vi "Find Device by Listbox Value.vi"(3 "error in (no error)":errorcluster, 4 "Listbox":refnum<vi>, 5 "ACNET Devices":refnum<class "ACNET Devices.lvclass">) -> (0 "error out":errorcluster, 1 "Found?":bool, 2 "ACNET Device Cluster":T1)   [LabVIEW 2013, in "ACNET Monitor.lvlib"]
uses:
  ACNET Monitor.lvlib
  ACNET Devices.lvclass
  ACNET Device.lvclass
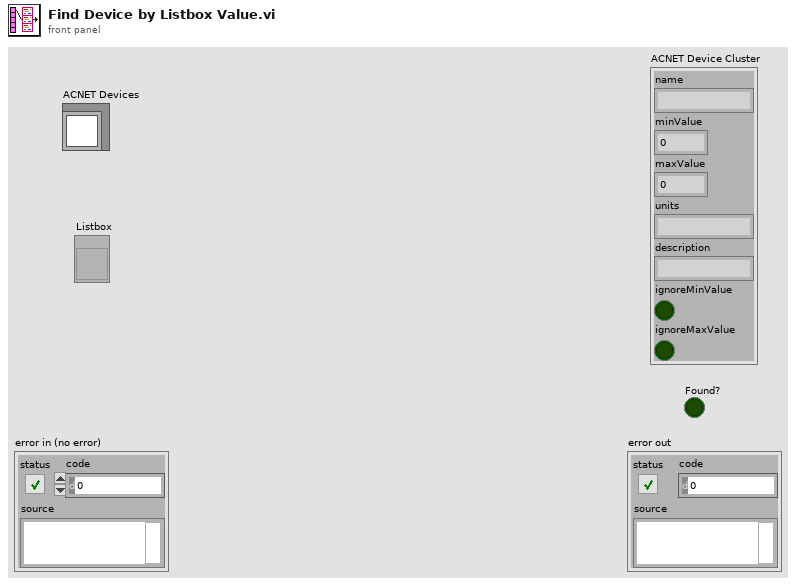
[diagram p1: front panel]
types:
  T1 = cluster{"name":string, "minValue":dbl, "maxValue":dbl, "units":string, "description":string, "ignoreMinValue":bool, "ignoreMaxValue":bool}
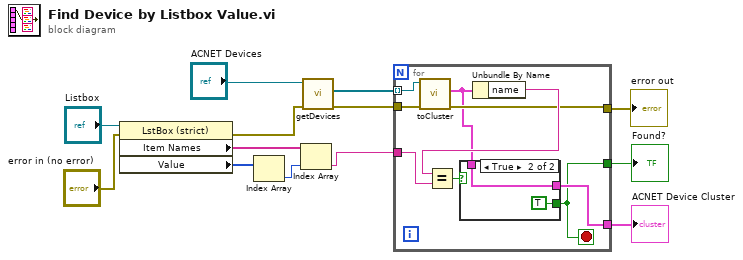
[diagram p0: block diagram]
diagram:
  n1 = property on="Property Node" class="LstBox (strict)"(reference="Listbox", error in="error in (no error)") -> (error out=w8:errorcluster, "Item Names"=w11:string[], "Value"=w5:i32[])  [unwired: 1 out]
  n2 = Index Array(array=w5) -> (element=w12:i32)  [unwired: 1 in]
  n3 = Index Array(array=w11, index=w12) -> (element=w13:string)
  n4 = call-dynamic "getDevices.vi"("error in (no error)"=w8, "ACNET Devices in"="ACNET Devices") -> ("error out"=w10:errorcluster, "Devices"=w9:refnum<class "ACNET Device.lvclass">[])  [unwired: 7 in, 1 out]
  n5 = for {
    tunnel: w9 -> [w22] mode=indexing
    tunnel: w10 -> [w21]
    tunnel: w13 -> [w19]
    tunnel: [w17] -> w3
    tunnel: [w15] -> w1
    tunnel: [w14] -> w2
    stop <- w14 stop-if-true
    n6 = call-dynamic "toCluster.vi"("error in (no error)"=w21, "ACNET Device in"=w22) -> ("error out"=w17:errorcluster, "ACNET Device Cluster"=w16:T1)  [unwired: 7 in, 1 out]
    n7 = Unbundle By Name(w16) -> ("name"=w20:string)
    n8 = Equal?(x=w20, y=w19) -> (x = y?=w18:bool)
    n9 = case shown="True" w18 {
      tunnel: [_ TRUE] -> w14
      tunnel: w16 -> [_ w23]
      tunnel: [_ w23] -> w15
      frame False {
      }
      frame True {
      }
    }
  }
  "error out" <- w3
  "Found?" <- w2
  "ACNET Device Cluster" <- w1
